vi "Manage Drive Ramp.vi"(11 "Drive Train Metrics Out in":T1) -> (3 "Drive Train Metrics Out out":T1)   [LabVIEW 2014]
uses:
  Drive Train Metrics.ctl
  CmdFlag.ctl
  DriveCals.vi
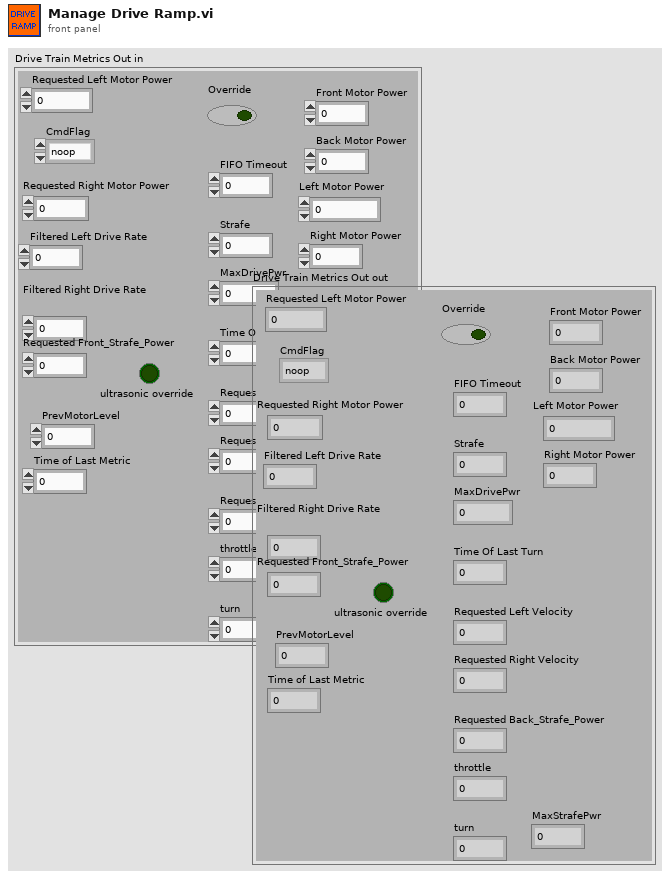
[diagram p1: front panel]
types:
  T1 = typedef "Drive Train Metrics.ctl" = cluster{"CmdFlag":T2, "Requested Right Motor Power":dbl, "Requested Left Motor Power":dbl, "Filtered Left Drive Rate":dbl, "Filtered Right Drive Rate":dbl, "Time of Last Metric":u32, "FIFO Timeout":i32, "Requested Left Velocity":dbl, "Requested Right Velocity":dbl, "throttle":dbl, "turn":dbl, "MaxDrivePwr":dbl, "Strafe":dbl, "Override":bool, "Time Of Last Turn":dbl, "Requested Front_Strafe_Power":dbl, "Requested Back_Strafe_Power":dbl, "MaxStrafePwr":dbl, "PrevMotorLevel":u8, "ultrasonic override":bool, "Left Motor Power":dbl, "Right Motor Power":dbl, "Front Motor Power":dbl, "Back Motor Power":dbl}
  T2 = typedef "CmdFlag.ctl" = enum16{"noop", "logflag", "suspend", "resume"}
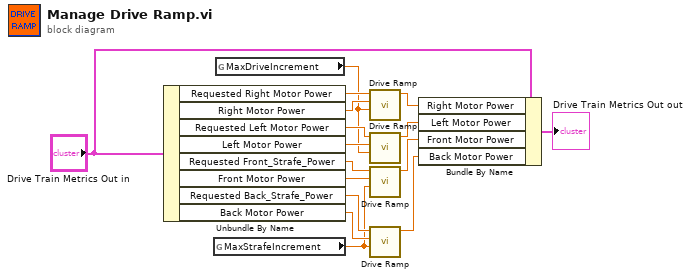
[diagram p0: block diagram]
diagram:
  n1 = Unbundle By Name("Drive Train Metrics Out in") -> ("Requested Right Motor Power"=w16:dbl, "Right Motor Power"=w15:dbl, "Requested Left Motor Power"=w11:dbl, "Left Motor Power"=w10:dbl, "Requested Front_Strafe_Power"=w8:dbl, "Front Motor Power"=w7:dbl, "Requested Back_Strafe_Power"=w4:dbl, "Back Motor Power"=w2:dbl)
  n2 = global read "DriveCals.vi" "MaxStrafeIncrement"() -> (w1:dbl)
  n3 = global read "DriveCals.vi" "MaxDriveIncrement"() -> (w3:dbl)
  n4 = call "Drive Ramp.vi"("MaxDriveIncrement"=w3, "Motor Power"=w15, "Requested  Motor Power in"=w16) -> ("Requested  Motor Power out"=w14:dbl)  [unwired: 8 in]
  n5 = call "Drive Ramp.vi"("MaxDriveIncrement"=w3, "Motor Power"=w10, "Requested  Motor Power in"=w11) -> ("Requested  Motor Power out"=w9:dbl)  [unwired: 8 in]
  n6 = call "Drive Ramp.vi"("MaxDriveIncrement"=w1, "Motor Power"=w7, "Requested  Motor Power in"=w8) -> ("Requested  Motor Power out"=w6:dbl)  [unwired: 8 in]
  n7 = call "Drive Ramp.vi"("MaxDriveIncrement"=w1, "Motor Power"=w2, "Requested  Motor Power in"=w4) -> ("Requested  Motor Power out"=w5:dbl)  [unwired: 8 in]
  n8 = Bundle By Name(cluster="Drive Train Metrics Out in", "Right Motor Power"=w14, "Left Motor Power"=w9, "Front Motor Power"=w6, "Back Motor Power"=w5) -> (→"Drive Train Metrics Out out":T1)
